vi "Resolve Relative URI.vi"(8 "error in (no error)":errorcluster, 10 "Base URI":refnum<class "URI.lvclass">, 11 "URI in":refnum<class "URI.lvclass">) -> (0 "error out":errorcluster, 3 "URI out":refnum<class "URI.lvclass">)   [LabVIEW 2020, in "Stream.lvlib" / "URI.lvclass"]
uses:
  URI.lvclass
  Stream.lvlib
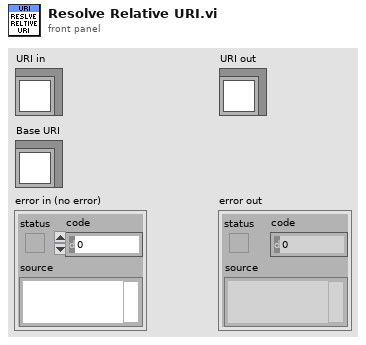
[diagram p1: front panel]
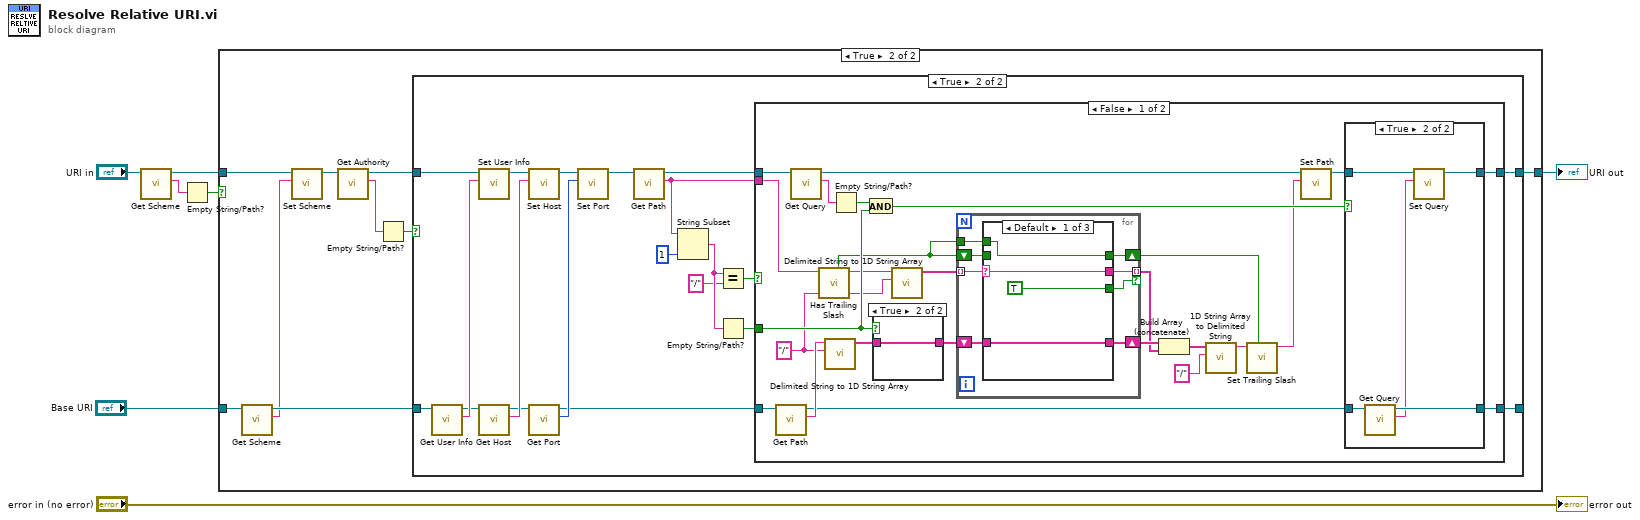
[diagram p0: block diagram]
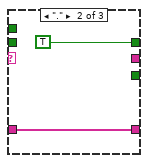
[diagram p4: hidden frame]
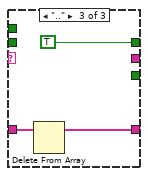
[diagram p5: hidden frame]
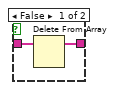
[diagram p6: hidden frame]
diagram:
  n1 = call "Get Scheme.vi"("URI in"="URI in") -> ("Scheme"=w2:string, "URI out"=w3:refnum<class "URI.lvclass">)  [unwired: 8 in, 1 out]
  n2 = Empty String/Path?(string/path=w2) -> (empty?=w1:bool)
  n3 = case shown="True" w1 {
    tunnel: "Base URI" -> [_ w14]
    tunnel: [w8 w9] -> w5
    tunnel: w3 -> [w8 w12]
    frame False {
    }
    frame True {
      n4 = call "Get Scheme.vi"("URI in"=w14) -> ("Scheme"=w10:string, "URI out"=w13:refnum<class "URI.lvclass">)  [unwired: 8 in, 1 out]
      n5 = call "Set Scheme.vi"("Scheme"=w10, "URI in"=w12) -> ("URI out"=w11:refnum<class "URI.lvclass">)  [unwired: 8 in, 1 out]
      n6 = call "Get Authority.vi"("URI in"=w11) -> ("Authority"=w17:string, "URI out"=w16:refnum<class "URI.lvclass">)  [unwired: 8 in, 1 out]
      n7 = Empty String/Path?(string/path=w17) -> (empty?=w15:bool)
      n8 = case shown="True" w15 {
        tunnel: w16 -> [w19 w38]
        tunnel: w13 -> [w18 w39]
        tunnel: [w18 w21] -> _
        tunnel: [w19 w20] -> w9
        frame False {
        }
        frame True {
          n9 = call "Get User Info.vi"("URI in"=w39) -> ("User Info"=w37:string, "URI out"=w36:refnum<class "URI.lvclass">)  [unwired: 8 in, 1 out]
          n10 = call "Set User Info.vi"("User Info"=w37, "URI in"=w38) -> ("URI out"=w35:refnum<class "URI.lvclass">)  [unwired: 8 in, 1 out]
          n11 = call "Get Host.vi"("URI in"=w36) -> ("Host"=w34:string, "URI out"=w33:refnum<class "URI.lvclass">)  [unwired: 8 in, 1 out]
          n12 = call "Set Host.vi"("Host"=w34, "URI in"=w35) -> ("URI out"=w32:refnum<class "URI.lvclass">)  [unwired: 8 in, 1 out]
          n13 = call "Get Port.vi"("URI in"=w33) -> ("Port"=w31:u16, "URI out"=w23:refnum<class "URI.lvclass">)  [unwired: 8 in, 1 out]
          n14 = call "Set Port.vi"("Port"=w31, "URI in"=w32) -> ("URI out"=w22:refnum<class "URI.lvclass">)  [unwired: 8 in, 1 out]
          n15 = call "Get Path.vi"("URI in"=w22) -> ("Path"=w28:string, "URI out"=w27:refnum<class "URI.lvclass">)  [unwired: 8 in, 1 out]
          n16 = String Subset(string=w28, length (rest)=1 ("length (rest)")) -> (substring=w30:string)  [unwired: 1 in]
          n17 = Equal?(x=w30, y="/") -> (x = y?=w26:bool)
          n18 = Empty String/Path?(string/path=w30) -> (empty?=w29:bool)
          n19 = case shown="False" w26 {
            tunnel: w23 -> [w65 w93]
            tunnel: w27 -> [w56 w94]
            tunnel: w28 -> [w44 _]
            tunnel: [w47 w94] -> w20
            tunnel: [w50 w93] -> w21
            tunnel: w29 -> [w53 _]
            frame False {
              w46 = "/" ("delimiter")
              n20 = call "Get Path.vi"("URI in"=w65) -> ("Path"=w64:string, "URI out"=w51:refnum<class "URI.lvclass">)  [unwired: 8 in, 1 out]
              n21 = call "Get Query.vi"("URI in"=w56) -> ("Query"=w55:string, "URI out"=w52:refnum<class "URI.lvclass">)  [unwired: 8 in, 1 out]
              n22 = call "Has Trailing Slash.vi"("Path In"=w44) -> ("Path"=w45:string, "Trailing Slash?"=w43:bool)  [unwired: 9 in]
              n23 = call <vilib>:"Delimited String to 1D String Array.vi"("delimiter"=w46, "delimited string"=w64) -> ("string array"=w62:string[])  [unwired: 9 in]
              n24 = Empty String/Path?(string/path=w55) -> (empty?=w54:bool)
              n25 = And(x=w54, y=w53) -> (x .and. y?=w49:bool)
              n26 = case shown="True" w53 {
                tunnel: w62 -> [w84 w85]
                tunnel: [w83 w85] -> w61
                frame False {
                  n27 = Delete From Array(array=w84) -> (array with subset deleted=w83:string[])  [unwired: 2 in, 1 out]
                }
                frame True {
                }
              }
              n28 = call <vilib>:"Delimited String to 1D String Array.vi"("delimiter"=w46, "delimited string"=w45) -> ("string array"=w63:string[])  [unwired: 9 in]
              n29 = for {
                tunnel: w63 -> [w73] mode=indexing
                shift-right: [w69] -> w60
                shift-left: w61 -> [w72]
                tunnel: [w71] -> w59 mode=indexing if=w70
                shift-right: [w67] -> w41
                shift-left: w43 -> [w68]
                tunnel: w43 -> [w66]
                n30 = case shown="Default" w73 {
                  selector: w73 -> [w77 _ _]
                  tunnel: w72 -> [w75 w79 w82]
                  tunnel: [w77 _ _] -> w71
                  tunnel: [TRUE _ _] -> w70
                  tunnel: [w75 w79 w81] -> w69
                  tunnel: w68 -> [_ _ _]
                  tunnel: [w74 TRUE TRUE ("Trailing Slash?")] -> w67
                  tunnel: w66 -> [w74 _ _]
                  frame Default {
                  }
                  frame "." {
                  }
                  frame ".." {
                    n31 = Delete From Array(array=w82) -> (array with subset deleted=w81:string[])  [unwired: 2 in, 1 out]
                  }
                }
              }
              n32 = Build Array (concatenate)(w60, w59) -> (w58:string[])
              n33 = call <vilib>:"1D String Array to Delimited String.vi"("delimiter"="/", "string array"=w58) -> ("delimited string"=w42:string)  [unwired: 9 in]
              n34 = call "Set Trailing Slash.vi"("Trailing Slash"=w41, "Path In"=w42) -> ("Path"=w40:string)  [unwired: 9 in]
              n35 = call "Set Path.vi"("Path"=w40, "URI in"=w52) -> ("URI out"=w48:refnum<class "URI.lvclass">)  [unwired: 8 in, 1 out]
              n36 = case shown="True" w49 {
                tunnel: w51 -> [w86 w92]
                tunnel: [w86 w91] -> w50
                tunnel: w48 -> [w87 w90]
                tunnel: [w87 w89] -> w47
                frame False {
                }
                frame True {
                  n37 = call "Get Query.vi"("URI in"=w92) -> ("Query"=w88:string, "URI out"=w91:refnum<class "URI.lvclass">)  [unwired: 8 in, 1 out]
                  n38 = call "Set Query.vi"("Query"=w88, "URI in"=w90) -> ("URI out"=w89:refnum<class "URI.lvclass">)  [unwired: 8 in, 1 out]
                }
              }
            }
            frame True {
            }
          }
        }
      }
    }
  }
  "URI out" <- w5
  "error out" <- "error in (no error)"
